vi "Measurement Logic.vi"() -> ()   [LabVIEW 2024, in "Pure Tone Generation (N Ch).lvlib"]
uses:
  Pure Tone Generation (N Ch).lvlib
  Measurement Results.ctl
  <vilib>/DAQmx/create/channels.llb/DAQmx Create Channel (AO-FuncGen).vi
  <vilib>/Plug-In SDKs/Measurements/Measure Call Context/Measure Call Context.lvclass
  Measurement Configuration.ctl
panel:
  out "measurement results":T1={"error out"=FALSE, "error description out"="Empty", "error code out"=0}
  in  "measurement configuration":T2={"physical channels"=["Lorem ipsum dolor sit", "Lorem ipsum dolor sit"], "frequencies"=[32.0, 33.0], "amplitudes"=[0.0, 0.0], "offsets"=[64.0, 65.0]}
  out "measure call context out":refnum<class "Measure Call Context.lvclass">
  in  "measure call context in":refnum<class "Measure Call Context.lvclass">
  out "error out":errorcluster
  in  "error in":errorcluster
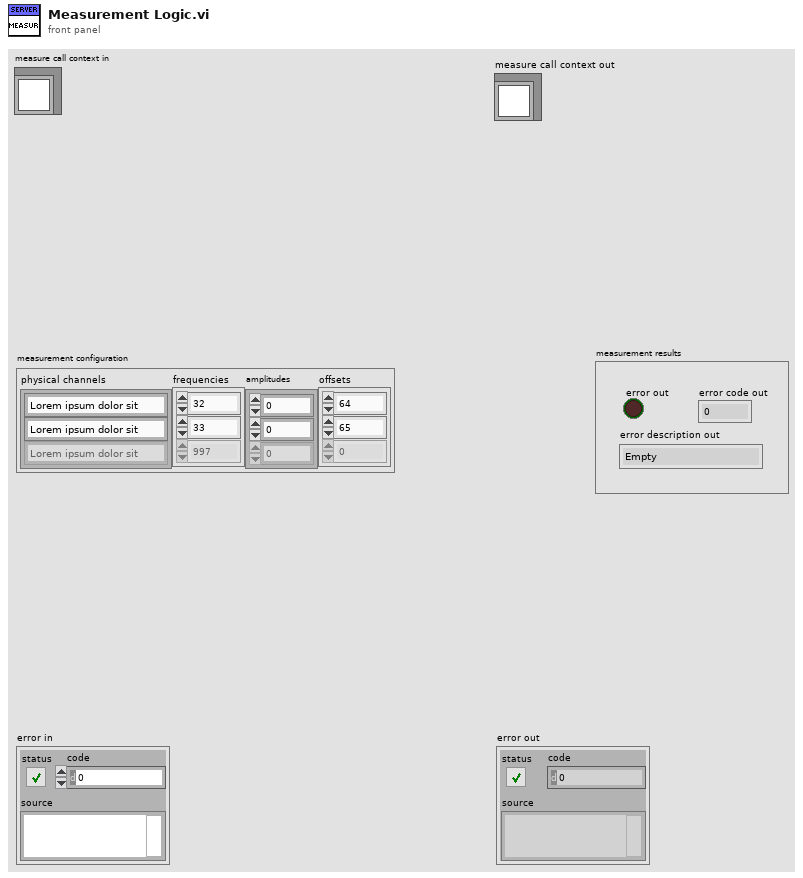
[diagram p1: front panel]
types:
  T1 = typedef "Pure Tone Generation (N Ch).lvlib/Measurement Results.ctl" = cluster{"error out":bool, "error description out":string, "error code out":i32}
  T2 = typedef "Pure Tone Generation (N Ch).lvlib/Measurement Configuration.ctl" = cluster{"physical channels":string[], "frequencies":dbl[], "amplitudes":dbl[], "offsets":dbl[]}
  T3 = typedef "Event Messenger-bool.lvlib/))Channel.ctl" = refnum<queue>
  T4 = typedef "Tag-bool.lvlib/))Channel.ctl" = refnum<queue>
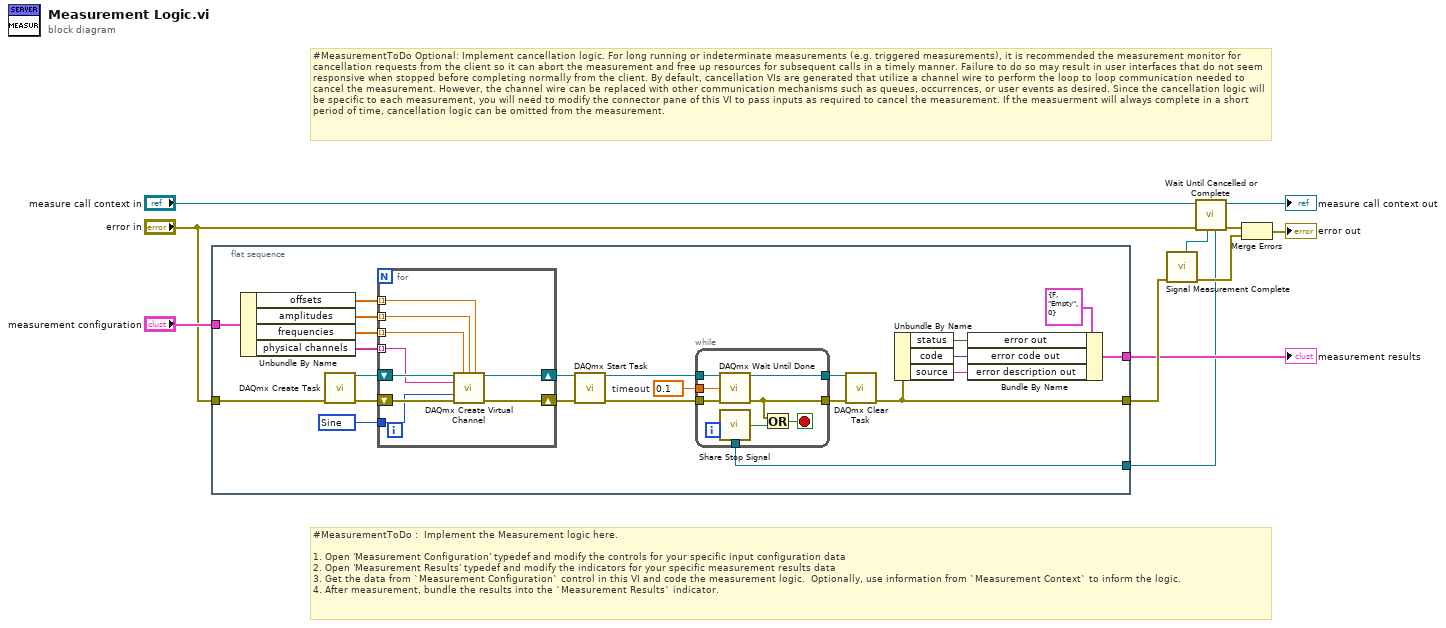
[diagram p0: block diagram]
diagram:
  # "#MeasurementToDo Optional: Implement cancellation logic. For long running or indeterminate measurements (e.g. triggered measurements), it is recommended the measurement monitor for cancellation requests from the client so it can abort the measurement and free up resources for subsequent calls in a timely manner. Failure to do so may result in user interfaces that do not seem responsive when stopped before completing normally from the client. By default, cancellation VIs are generated that utilize a channel wire to perform the loop to loop communication needed to cancel the measurement. However, the channel wire can be replaced with other communication mechanisms such as queues, occurrences, or user events as desired. Since the cancellation logic will be specific to each measurement, you will need to modify the connector pane of this VI to pass inputs as required to cancel the measurement. If the measuerment will always complete in a short period of time, cancellation logic can be omitted from the measurement."
  # "#MeasurementToDo :  Implement the Measurement logic here.\n\n1. Open 'Measurement Configuration' typedef and modify the controls for your specific input configuration data\n2. Open 'Measurement Results' typedef and modify the indicators for your specific measurement results data\n3. Get the data from `Measurement Configuration` control in this VI and code the measurement logic.  Optionally, use information from `Measurement Context` to inform the logic.\n4. After measurement, bundle the results into the `Measurement Results` indicator."
  n1 = flat-sequence {
    tunnel: "measurement configuration" -> [w17]
    tunnel: "error in" -> [w26]
    tunnel: [w22] -> w7
    tunnel: [w18] -> w2
    tunnel: w1 -> [w12]
    frame #0 {
      w24 = 0.1  # timeout
      w25 = 14751 items=["Sine"=14751, "Triangle"=14752, "Square"=14753, "Sawtooth"=14754] ("type")
      n2 = Unbundle By Name(w17) -> ("offsets"=w13:dbl[], "amplitudes"=w14:dbl[], "frequencies"=w15:dbl[], "physical channels"=w16:string[])
      n3 = call <vilib>:"DAQmx Create Task.vi"("error in"=w26) -> ("task out"=w34:refnum<k21>, "error out"=w33:errorcluster)  [unwired: 13 in]
      n4 = for {
        shift-right: [w51] -> w32
        shift-left: w34 -> [w50]
        shift-right: [w48] -> w31
        shift-left: w33 -> [w49]
        tunnel: w25 -> [w47]
        tunnel: w16 -> [w46] mode=indexing
        tunnel: w15 -> [w45] mode=indexing
        tunnel: w14 -> [w44] mode=indexing
        tunnel: w13 -> [w43] mode=indexing
        n5 = call-poly <vilib>:"DAQmx Create Virtual Channel.vi"("task in"=w50, "frequency"=w45, "amplitude"=w44, "offset"=w43, "physical channels"=w46, "type"=w47, "error in"=w49) -> ("task out"=w51:refnum<k21>, "error out"=w48:errorcluster)  [unwired: 7 in]
      }
      n6 = call <vilib>:"DAQmx Start Task.vi"("task/channels in"=w32, "error in"=w31) -> ("task out"=w30:refnum<k21>, "error out"=w29:errorcluster)  [unwired: 12 in]
      n7 = while {
        tunnel: w30 -> [w42]
        tunnel: w29 -> [w41]
        tunnel: [w40] -> w28
        tunnel: [w39] -> w27
        tunnel: w24 -> [w37]
        tunnel: w12 -> [w36]
        stop <- w38 stop-if-true
        n8 = call <vilib>:"DAQmx Wait Until Done.vi"("task/channels in"=w42, "timeout (sec)"=w37, "error in"=w41) -> ("task out"=w40:refnum<k21>, "error out"=w39:errorcluster)  [unwired: 11 in]
        n9 = call <vilib>:"Share Stop Signal.vi"("channel"=w36) -> ("stop"=w35:bool)  [unwired: 1 in]
        n10 = Or(x=w39, y=w35) -> (x .or. y?=w38:bool)
      }
      n11 = call <vilib>:"DAQmx Clear Task.vi"("task in"=w28, "error in"=w27) -> ("error out"=w22:errorcluster)  [unwired: 13 in]
      n12 = Unbundle By Name(w22) -> ("status"=w21:bool, "code"=w20:i32, "source"=w19:string)
      n13 = Bundle By Name(cluster=T1 {"error out"=FALSE, "error description out"="Empty", "error code out"=0} ("Measurement Results"), "error out"=w21, "error code out"=w20, "error description out"=w19) -> (w18:T1)
    }
  }
  n14 = call "Signal Measurement Complete.vi"("error in (no error)"=w7) -> ("error out"=w5:errorcluster, "done channel"=w6:T3)  [unwired: 9 in]
  n15 = call "Wait Until Cancelled or Complete.vi"("done channel"=w6, "error in (no error)"="error in", "measure call context in"="measure call context in") -> ("error out"=w4:errorcluster, "measure call context out"=→"measure call context out":refnum<class "Measure Call Context.lvclass">, "stop channel"=w1:T4)  [unwired: 6 in]
  n16 = Merge Errors(w4, w5) -> (→"error out":errorcluster)
  "measurement results" <- w2
